vi "OPC.vi"() -> ()   [LabVIEW 2018]
uses:
  05.UserVI's/file io/ini/type defs/ini entry value.ctl
  05.UserVI's/file io/ini/type defs/ini entry.ctl
  05.UserVI's/file io/ini/type defs/ini entry types.ctl
  05.UserVI's/file io/ini/type defs/ini file actions.ctl
panel:
  out "数组":string[](array[string])
  out "values out":T1[](array[typedef])
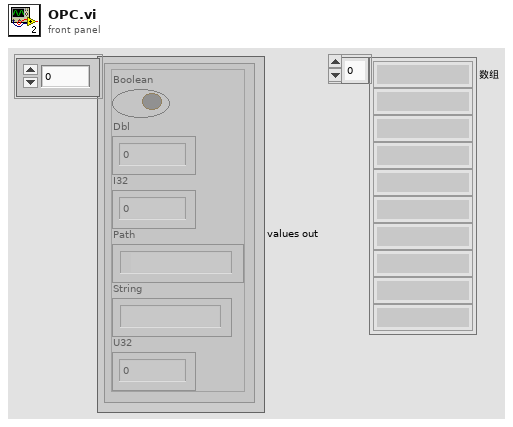
[diagram p1: front panel]
types:
  T1 = typedef "ini entry value.ctl" = cluster{"Boolean":bool, "Dbl":dbl, "I32":i32, "Path":path, "String":string, "U32":u32}
  T2 = typedef "ini file actions.ctl" = enum16{"read ini", "write ini"}
  T3 = typedef "ini entry.ctl" = cluster{"section":string, "key":string, "type":T4, "default value":T1}
  T4 = typedef "ini entry types.ctl" = enum16{"Boolean", "Double", "I32", "Path", "String", "U32"}
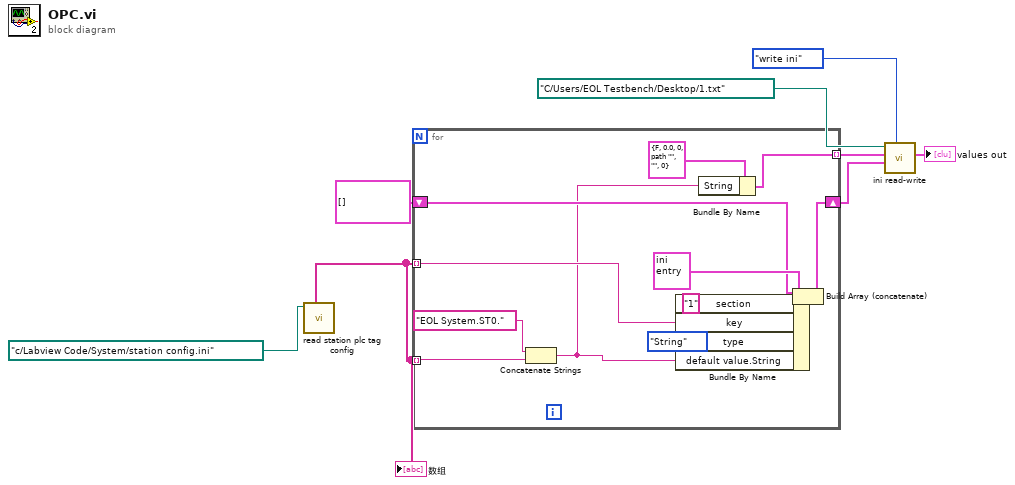
[diagram p0: block diagram]
diagram:
  n1 = call "read station plc tag config.vi"("configuration file path in"=path "c:/Labview Code/System/station config.ini" ("station config file path")) -> ("数组"=w1:string[])  [unwired: 7 in, 3 out]
  "数组" <- w1
  n2 = for {
    tunnel: w1 -> [w19] mode=indexing
    shift-right: [w16] -> w7
    shift-left: T3[] [] -> [w15]
    tunnel: w1 -> [w11] mode=indexing
    tunnel: [w12] -> w3 mode=indexing
    n3 = Concatenate Strings("EOL System.ST0." ("字符串"), w11) -> (w9:string)
    n4 = Bundle By Name(cluster=T3 {"section"="", "key"="", "type"=enum."Boolean", "default value"={"Boolean"=FALSE, "Dbl"=0.0, "I32"=0, "Path"=path "", "String"="", "U32"=0}}, "section"="1", "key"=w19, "type"=ini_entry_types."String", "default value.String"=w9) -> (w14:T3)
    n5 = Bundle By Name(cluster=T1 {"Boolean"=FALSE, "Dbl"=0.0, "I32"=0, "Path"=path "", "String"="", "U32"=0}, "String"=w9) -> (w12:T1)
    n6 = Build Array (concatenate)(w15, w14) -> (w16:T3[])
  }
  n7 = call "ini read-write.vi"("action"=ini_file_actions."write ini", "ini entry descriptors"=w7, "values in"=w3, "configuration file path"=path "C:/Users/EOL Testbench/Desktop/1.txt") -> ("values out"=→"values out":T1[])  [unwired: 5 in, 2 out]
